vi "Read age.vi"(8 "error in (no error)":errorcluster, 11 "myClass in":refnum<class "myClass.lvclass">) -> (0 "error out":errorcluster, 2 "age":dbl, 3 "myClass out":refnum<class "myClass.lvclass">)   [LabVIEW 2009, in "myClass.lvclass"]
uses:
  myClass.lvclass
  myClass.lvclass/myClass.ctl
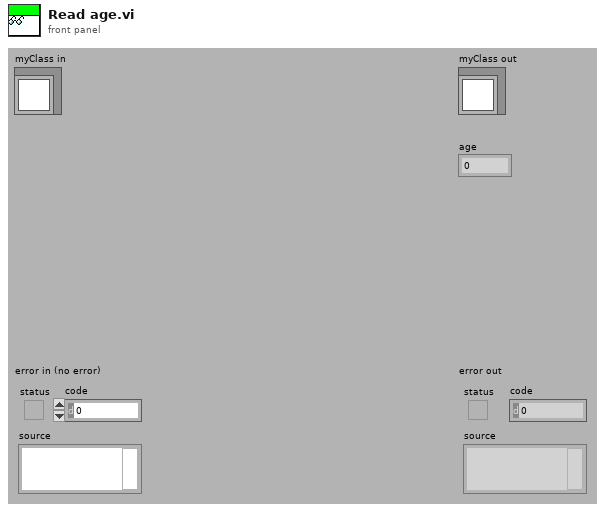
[diagram p1: front panel]
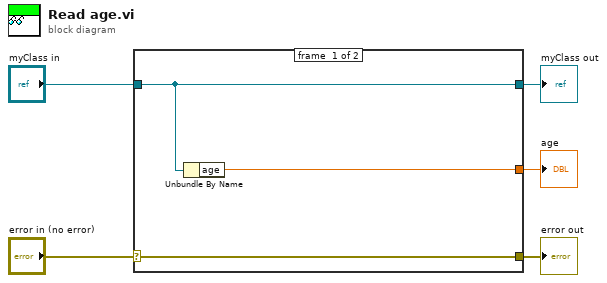
[diagram p0: block diagram]
diagram:
  n1 = case shown="No Error" "error in (no error)" {
    selector: "error in (no error)" -> [w8 w9]
    tunnel: [w8 w9] -> w4
    tunnel: [w7 w10] -> w2
    tunnel: "myClass in" -> [w7 w10]
    tunnel: [w6 _] -> w1
    frame #0 {
      n2 = Unbundle By Name(w7) -> ("age"=w6:dbl)
    }
    frame #1 {
    }
  }
  "error out" <- w4
  "myClass out" <- w2
  "age" <- w1
